vi "Change Win Shell.vi"(4 "error in (no error)":errorcluster, 7 "New Shell Path":path) -> (0 "error out":errorcluster, 3 "Old Shell Path":path)   [LabVIEW 2011]
uses:
  <vilib>/registry/registry.llb/Registry RtKey.ctl
  <vilib>/registry/registry.llb/Read Registry Value Simple STR.vi
  <vilib>/registry/registry.llb/Write Registry Value Simple STR.vi
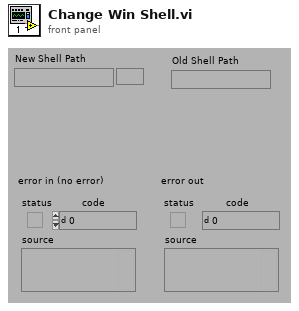
[diagram p1: front panel]
types:
  T1 = typedef "Registry RtKey.ctl" = enum32{"HKEY_CLASSES_ROOT", "HKEY_CURRENT_USER", "HKEY_LOCAL_MACHINE", "HKEY_USERS", "HKEY_PERFORMANCE_DATA", "HKEY_CURRENT_CONFIG", "HKEY_DYN_DATA"}
  T2 = typedef "Registry refnum.ctl" = refnum<k1>
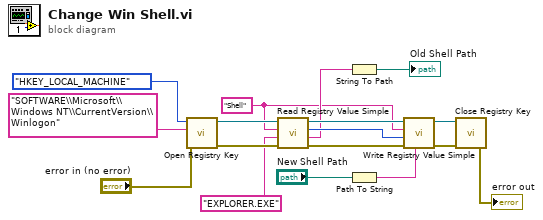
[diagram p0: block diagram]
diagram:
  w2 = "Shell"
  n1 = call <vilib>:"Open Registry Key.vi"("error in (no error)"="error in (no error)", "subkey"="SOFTWARE\\Microsoft\\Windows NT\\CurrentVersion\\Winlogon", "root key (HKEY_LOCAL_MACHINE)"=Registry_RtKey."HKEY_LOCAL_MACHINE") -> ("error out"=w9:errorcluster, "refnum out"=w10:T2)  [unwired: 7 out]
  n2 = call-poly <vilib>:"Read Registry Value Simple.vi"("error in (no error)"=w9, "default data"="EXPLORER.EXE", "value"=w2, "refnum"=w10) -> ("error out"=w8:errorcluster, "String/Binary data"=w6:string, "simple data type"=w7:enum16{"String", "Binary", "DWORD"}, "refnum out"=w11:T2)  [unwired: 2 out]
  n3 = String To Path(string=w6) -> (path=→"Old Shell Path":path)
  n4 = Path To String(path="New Shell Path") -> (string=w13:string)
  n5 = call-poly <vilib>:"Write Registry Value Simple.vi"("String/Binary data"=w13, "error in (no error)"=w8, "simple data type"=w7, "value"=w2, "refnum"=w11) -> ("error out"=w15:errorcluster, "refnum out"=w14:T2)  [unwired: 3 out]
  n6 = call <vilib>:"Close Registry Key.vi"("error in (no error)"=w15, "refnum"=w14) -> ("error out"=→"error out":errorcluster)  [unwired: 5 out]
